vi "Configure Calibration Factors.vi"(8 "error in (no error)":errorcluster, 10 "calibration factors":dbl[](array[numeric]), 11 "VGC in":refnum<class "PL Inficon VGC.lvclass">) -> (0 "error out":errorcluster, 2 "calibration factors":dbl[](array[numeric]), 3 "VGC out":refnum<class "PL Inficon VGC.lvclass">)   [LabVIEW 2015, in "PL Inficon VGC.lvclass"]
doc: "Configures calibration factors."
uses:
  PL Inficon VGC.lvclass
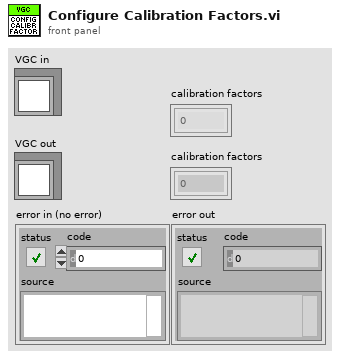
[diagram p1: front panel]
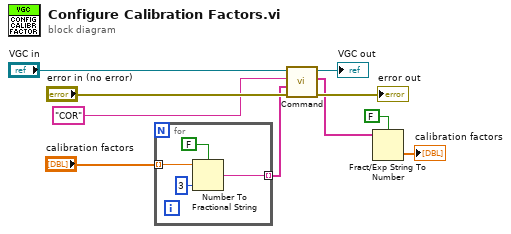
[diagram p0: block diagram]
diagram:
  n1 = for {
    tunnel: "calibration factors" -> [w12] mode=indexing
    tunnel: [w11] -> w3 mode=indexing
    n2 = Number To Fractional String(use system decimal point (T)=FALSE, number=w12, precision (6)=i16 3) -> (F-format string=w11:string)  [unwired: 1 in]
  }
  n3 = call "Command.vi"("error in (no error)"="error in (no error)", "parameters"=w3, "command"="COR" ("format string"), "VGC in"="VGC in") -> ("error out"=→"error out":errorcluster, "response data"=w2:string[], "VGC out"=→"VGC out":refnum<class "PL Inficon VGC.lvclass">)  [unwired: 5 in]
  n4 = Fract/Exp String To Number(use system decimal point (T)=FALSE, string=w2) -> (number=→"calibration factors":dbl[])  [unwired: 2 in, 1 out]
